vi "excel写.vi"(0 "路径":path, 1 "Table":string[][](table)=[["1", "2", "3", "4", "5", "6", "7", "8", "9", "10"], ["10", "11", "12", "13", "14", "15", "16", "17", "18", "19"], ["20", "21", "22", "23", "24", "25", "26", "27", "28", "29"], ["30", "31", "32", "33", "34", "35", "36", "37", "38", "39"]], 2 "数值":i8) -> ()   [LabVIEW 2013]
doc: "This VI demonstrates the use of ActiveX to write a table into a Microsoft Excel worksheet."
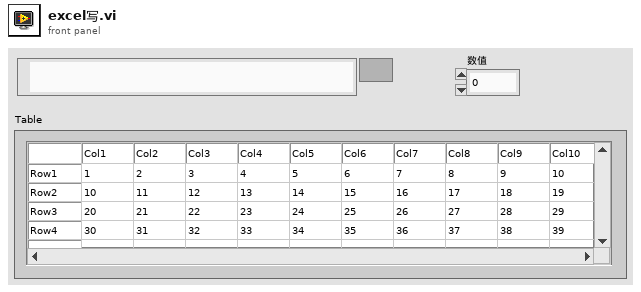
[diagram p1: front panel]
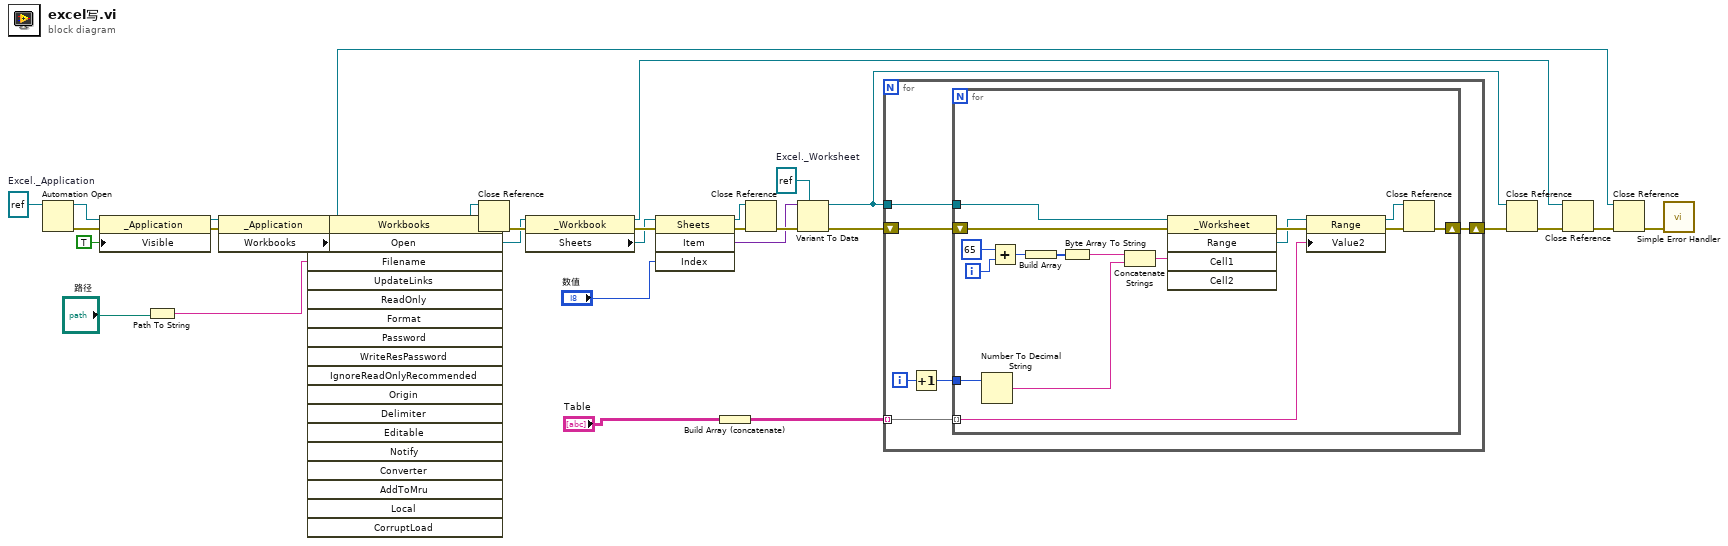
[diagram p0: block diagram]
diagram:
  w10 = refnum<k7> refnum  # Excel._Worksheet
  w26 = refnum<k7> refnum  # Excel._Application
  n1 = Automation Open(Automation Refnum=w26) -> (Automation Refnum=w27:refnum<k7>, error out=w28:errorcluster)  [unwired: 1 in, 2 out]
  n2 = property class="_Application"(reference=w27, error in=w28, "Visible"=TRUE) -> (reference out=w19:refnum<k7>, error out=w21:errorcluster)
  n3 = Path To String(path="路径") -> (string=w3:string)
  n4 = property class="_Application"(reference=w19, error in=w21) -> (reference out=w16:refnum<k7>, error out=w24:errorcluster, "Workbooks"=w25:refnum<k7>)
  n5 = invoke class="Workbooks" method="Open"(reference=w25, error in=w24, "Filename"=w3) -> (reference out=w22:refnum<k7>, error out=w23:errorcluster, "Open"=w17:refnum<k7>)  [unwired: 15 in, 15 out]
  n6 = Close Reference(reference=w22, error in (no error)=w23) -> (error out=w18:errorcluster)
  n7 = property class="_Workbook"(reference=w17, error in=w18) -> (reference out=w14:refnum<k7>, error out=w8:errorcluster, "Sheets"=w7:refnum<k7>)
  n8 = invoke class="Sheets" method="Item"(reference=w7, error in=w8, "Index"="数值") -> (reference out=w11:refnum<k7>, error out=w12:errorcluster, "Item"=w9:variant)  [unwired: 1 in, 1 out]
  n9 = Build Array (concatenate)("Table") -> (w1:string[][])
  n10 = Close Reference(reference=w11, error in (no error)=w12) -> (error out=w13:errorcluster)
  n11 = Variant To Data(error in=w13, type=w10, Variant=w9) -> (data=w15:refnum<k7>, error out=w6:errorcluster)
  n12 = for {
    shift-right: [w37] -> w29
    shift-left: w6 -> [w38]
    tunnel: w15 -> [w36]
    tunnel: w1 -> [w33] mode=indexing
    i -> [w35]
    n13 = Increment(x=w35) -> (x+1=w34:i32)
    n14 = for {
      shift-right: [w50] -> w37
      shift-left: w38 -> [w48]
      tunnel: w36 -> [w47]
      tunnel: w34 -> [w42]
      tunnel: w33 -> [w52] mode=indexing
      i -> [w43]
      n15 = Number To Decimal String(number=w42) -> (decimal integer string=w40:string)  [unwired: 1 in]
      n16 = Add(x=65, y=w43) -> (x+y=w45:i32)
      n17 = Build Array(w45) -> (w44:i32[])
      n18 = Byte Array To String(unsigned byte array=w44) -> (string=w41:string)
      n19 = Concatenate Strings(w41, w40) -> (w39:string)
      n20 = invoke class="_Worksheet" method="Range"(reference=w47, error in=w48, "Cell1"=w39) -> (error out=w54:errorcluster, "Range"=w53:refnum<k7>)  [unwired: 2 in, 3 out]
      n21 = property class="Range"(reference=w53, error in=w54, "Value2"=w52) -> (reference out=w49:refnum<k7>, error out=w51:errorcluster)
      n22 = Close Reference(reference=w49, error in (no error)=w51) -> (error out=w50:errorcluster)
    }
  }
  n23 = Close Reference(reference=w15, error in (no error)=w29) -> (error out=w32:errorcluster)
  n24 = Close Reference(reference=w14, error in (no error)=w32) -> (error out=w31:errorcluster)
  n25 = Close Reference(reference=w16, error in (no error)=w31) -> (error out=w30:errorcluster)
  n26 = call <vilib>:"Simple Error Handler.vi"("error in (no error)"=w30) -> ()  [unwired: 4 in, 5 out]
